vi "BallPositionTracking.vi"(8 "error in (no error)":errorcluster, 9 "Tracking treshold":i32=40, 10 "Circles Data":T2(array[cluster]), 11 "Screen Dimensions":cluster{"x":i32, "y":i32}) -> (0 "error out":errorcluster, 1 "maxDistance":i32, 2 "Ball Tracking Position Data":T1, 3 "Speed":i32, 5 "OOB":bool)   [LabVIEW 2015]
uses:
  <vilib>/vision/NI_Vision_Development_Module.lvlib
  <vilib>/Analysis/NI_AALPro.lvlib
panel:
  # "Input"
  # "Output"
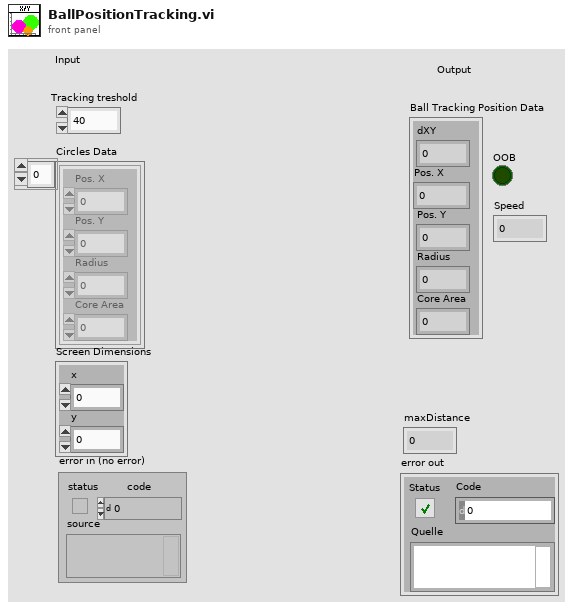
[diagram p1: front panel]
types:
  T1 = cluster{"dXY":i32, "Pos. X":i32, "Pos. Y":i32, "Radius":i32, "Core Area":i32}
  T2 = cluster{"Pos. X":i32, "Pos. Y":i32, "Radius":i32, "Core Area":i32}[]
  T3 = cluster{"dXY":i32, "Pos. X":i32, "Pos. Y":i32, "Radius":i32, "Core Area":i32}[]
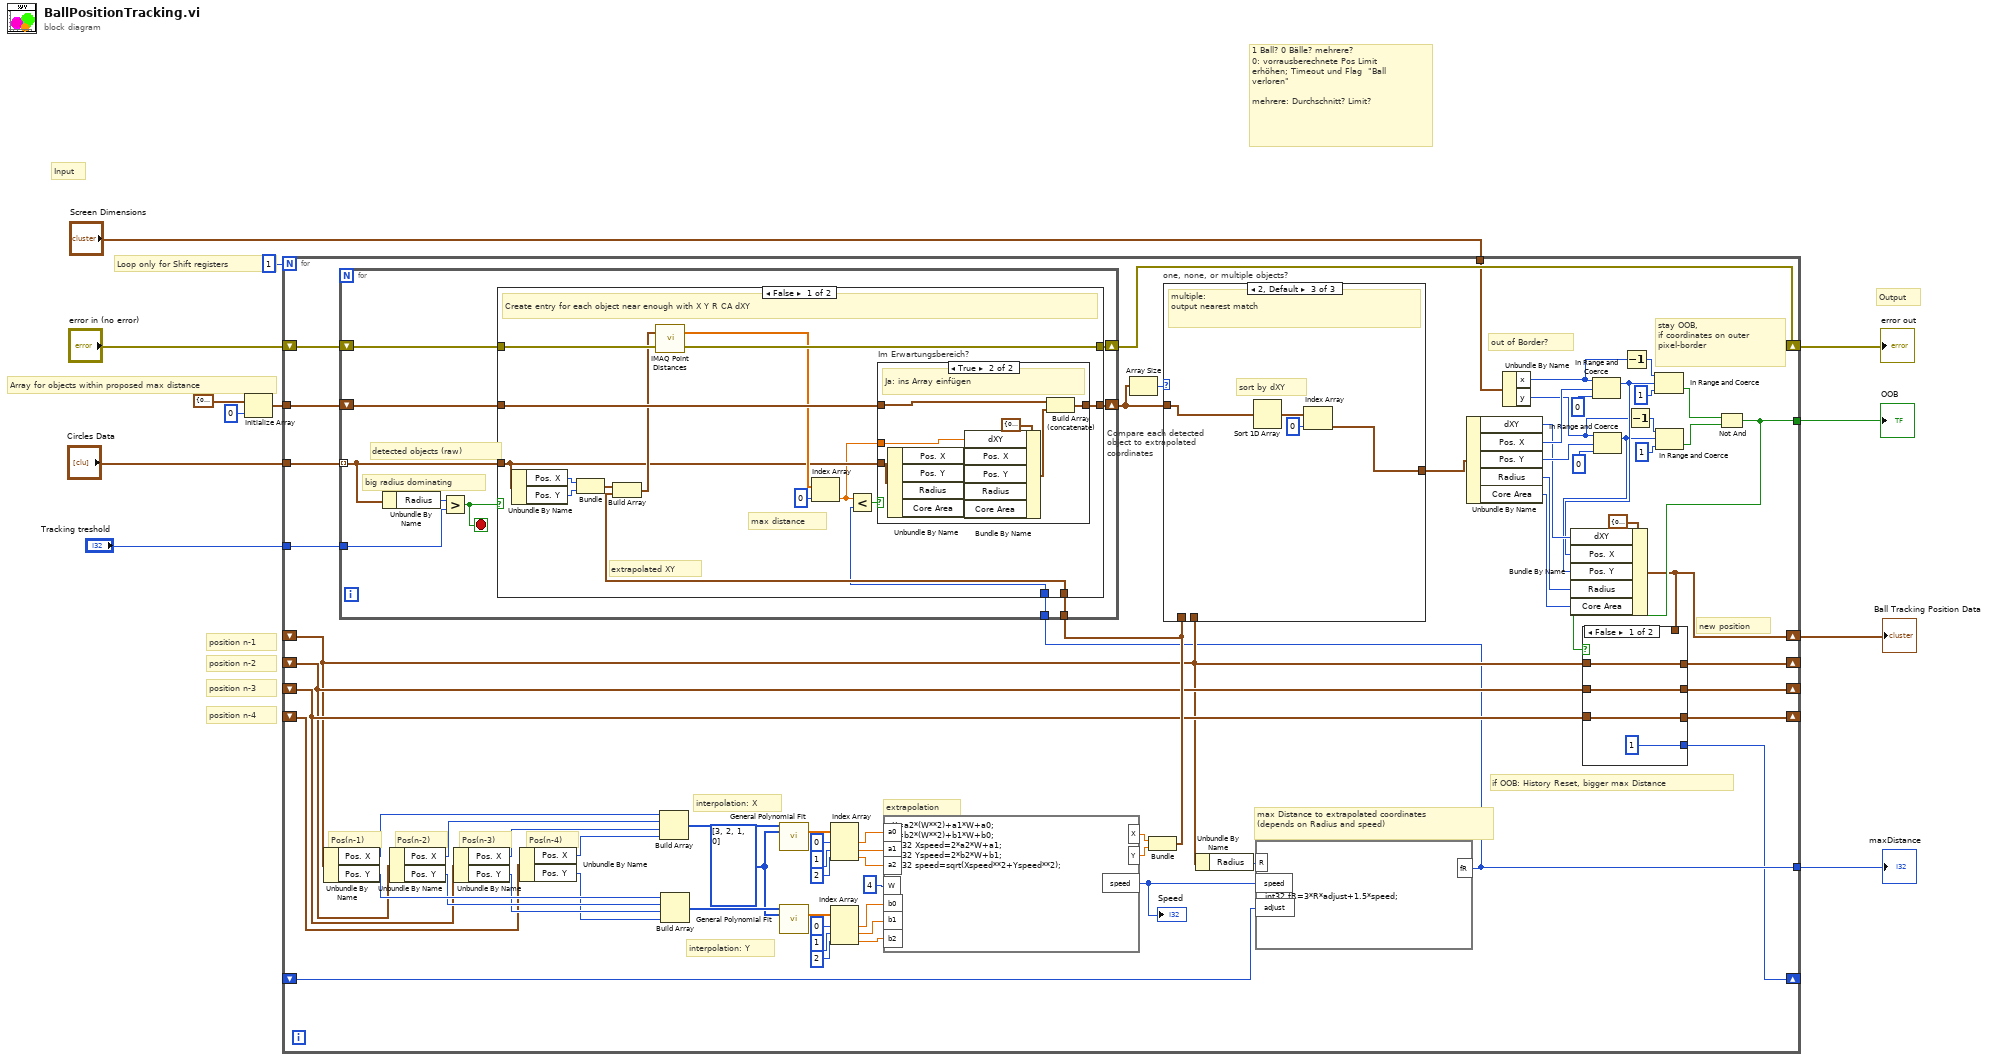
[diagram p0: block diagram]
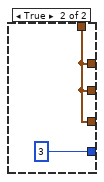
[diagram p2: hidden frame]
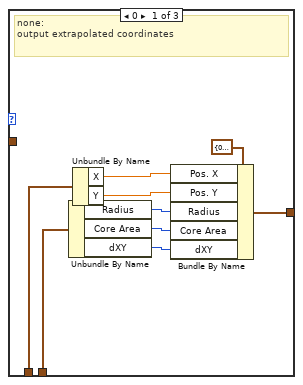
[diagram p3: hidden frame]
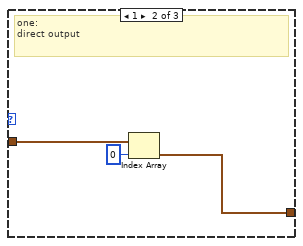
[diagram p4: hidden frame]
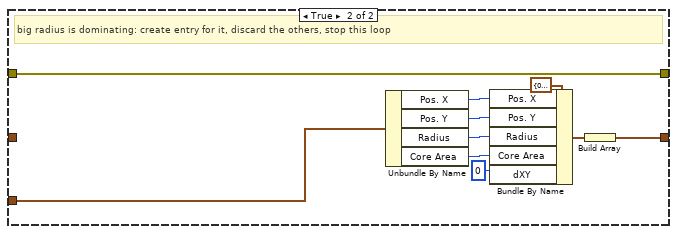
[diagram p6: hidden frame]
diagram:
  # "1 Ball? 0 Bälle? mehrere?\n0: vorrausberechnete Pos Limit erhöhen; Timeout und Flag  \"Ball verloren\"\n\nmehrere: Durchschnitt? Limit?"
  # "position n-4"
  # "Array for objects within proposed max distance"
  # "Loop only for Shift registers"
  # "position n-3"
  # "position n-2"
  # "position n-1"
  # "Output"
  # "Input"
  n1 = Initialize Array(T1 {"dXY"=0, "Pos. X"=0, "Pos. Y"=0, "Radius"=0, "Core Area"=0} ("Circles Data"), 0 ("Dimension")) -> (w8:T3)
  n2 = for {
    N: 1 -> [_]
    shift-right: [w30] -> w11
    shift-left: _ -> [w19]
    shift-right: [w80] -> w3
    shift-left: "error in (no error)" -> [w81]
    shift-right: [w34] -> _
    shift-left: _ -> [w35]
    shift-right: [w33] -> _
    shift-left: _ -> [w36]
    tunnel: w8 -> [w69]
    shift-right: [w32] -> _
    shift-left: _ -> [w49]
    tunnel: "Screen Dimensions" -> [w46]
    tunnel: [w31] -> w5
    tunnel: "Circles Data" -> [w82]
    tunnel: [w16] -> w4
    shift-right: [w14] -> _
    shift-left: _ -> [w15]
    tunnel: "Tracking treshold" -> [w13]
    w72 = i32[] [3, 2, 1, 0] ("X")
    # "new position"
    # "max Distance to extrapolated coordinates\n(depends on Radius and speed)"
    # "stay OOB,\nif coordinates on outer\npixel-border"
    # "if OOB: History Reset, bigger max Distance"
    # "out of Border?"
    # "Pos(n-4)"
    # "Pos(n-3)"
    # "Pos(n-2)"
    # "Pos(n-1)"
    # "extrapolation"
    # "interpolation: Y"
    # "interpolation: X"
    n3 = Unbundle By Name(w19) -> ("Pos. X"=w79:i32, "Pos. Y"=w76:i32)
    n4 = Unbundle By Name(w35) -> ("Pos. X"=w78:i32, "Pos. Y"=w75:i32)
    n5 = Unbundle By Name(w36) -> ("Pos. X"=w68:i32, "Pos. Y"=w74:i32)
    n6 = Unbundle By Name(w49) -> ("Pos. X"=w47:i32, "Pos. Y"=w48:i32)
    n7 = Build Array(w79, w78, w68, w47) -> (w77:i32[])
    n8 = Build Array(w76, w75, w74, w48) -> (w73:i32[])
    n9 = call <vilib>:"General Polynomial Fit.vi"("Y"=w77, "X"=w72) -> ("Polynomial Coefficients"=w54:dbl[])  [unwired: 10 in, 3 out]
    n10 = call <vilib>:"General Polynomial Fit.vi"("Y"=w73, "X"=w72) -> ("Polynomial Coefficients"=w64:dbl[])  [unwired: 10 in, 3 out]
    n11 = Index Array(array=w54, index #1=0 ("Index"), index #2=1 ("Index"), index #3=2 ("Index")) -> (element #1=w53:dbl, element #2=w52:dbl, element #3=w51:dbl)
    n12 = Index Array(array=w64, index #1=0 ("Index"), index #2=1 ("Index"), index #3=2 ("Index")) -> (element #1=w60:dbl, element #2=w59:dbl, element #3=w58:dbl)
    n13 = formula code="X=a2*(W**2)+a1*W+a0;\nY=b2*(W**2)+b1*W+b0;\nint32 Xspeed=2*a2*W+a1;\nint32 Yspeed=2*b2*W+b1;\nint32 speed=sqrt(Xspeed**2+Yspeed**2);"("a1"=w52, "b2"=w58, "a0"=w53, "b0"=w60, "b1"=w59, "a2"=w51, "W"=4 ("Eingangsvariable")) -> ("X"=w71:dbl, "Y"=w70:dbl, "speed"=w18:i32)
    "Speed" <- w18
    n14 = Bundle("X"=w71, "Y"=w70) -> (w65:cluster{"X":dbl, "Y":dbl})  [unwired: 1 in]
    n15 = Unbundle By Name(w19) -> ("Radius"=w17:i32)
    n16 = formula code="int32 fR=3*R*adjust+1.5*speed;"("R"=w17, "speed"=w18, "adjust"=w15) -> ("fR"=w16:i32)
    n17 = for {
      tunnel: w82 -> [w113] mode=indexing
      shift-right: [w109] -> w80
      shift-left: w81 -> [w110]
      tunnel: w65 -> [w111]
      shift-right: [w107] -> w66
      shift-left: w69 -> [w108]
      tunnel: w16 -> [w106]
      tunnel: w13 -> [w105]
      stop <- w112 stop-if-true
      # "detected objects (raw)"
      # "big radius dominating"
      n18 = Unbundle By Name(w113) -> ("Radius"=w114:i32)
      n19 = Greater?(x=w114, y=w105) -> (0:w112:bool)
      n20 = case "Compare each detected object to extrapolated coordinates" shown="False" w112 {
        tunnel: w113 -> [w118 w141]
        tunnel: w111 -> [w116 _]
        tunnel: w110 -> [w129 w150]
        tunnel: [w128 w150] -> w109
        tunnel: w108 -> [w124 _]
        tunnel: [w123 w142] -> w107
        tunnel: w106 -> [w115 _]
        frame False {
          # "max distance"
          # "extrapolated XY"
          # "Create entry for each object near enough with X Y R CA dXY"
          n21 = Unbundle By Name(w118) -> ("Pos. X"=w126:i32, "Pos. Y"=w125:i32)
          n22 = Bundle("Pos. X"=w126, "Pos. Y"=w125) -> (w127:cluster{"Pos. X":i32, "Pos. Y":i32})  [unwired: 1 in]
          n23 = Build Array(w127, w116) -> (w121:cluster{"X":dbl, "Y":dbl}[])
          n24 = call "IMAQ Point Distances"("Points"=w121, "error in (no error)"=w129) -> ("Distances"=w119:sgl[], "error out"=w128:errorcluster)  [unwired: 3 in]
          n25 = Index Array(array=w119, index=0 ("Index")) -> (element=w117:sgl)
          n26 = Less?(x=w117, y=w115) -> (x < y?=w122:bool)
          n27 = case "Im Erwartungsbereich?" shown="True" w122 {
            tunnel: w124 -> [w130 w140]
            tunnel: [w130 w137] -> w123
            tunnel: w118 -> [_ w139]
            tunnel: w117 -> [_ w131]
            frame False {
              # "Nein: nicht hinzufügen"
            }
            frame True {
              # "Ja: ins Array einfügen"
              n28 = Unbundle By Name(w139) -> ("Pos. X"=w135:i32, "Pos. Y"=w134:i32, "Radius"=w133:i32, "Core Area"=w132:i32)
              n29 = Bundle By Name(cluster=T1 {"dXY"=0, "Pos. X"=0, "Pos. Y"=0, "Radius"=0, "Core Area"=0} ("Circles Data"), "dXY"=w131, "Pos. X"=w135, "Pos. Y"=w134, "Radius"=w133, "Core Area"=w132) -> (w136:T1)
              n30 = Build Array (concatenate)(w140, w136) -> (w137:T3)
            }
          }
        }
        frame True {
          # "big radius is dominating: create entry for it, discard the others, stop this loop"
          n31 = Unbundle By Name(w141) -> ("Pos. X"=w148:i32, "Pos. Y"=w147:i32, "Radius"=w146:i32, "Core Area"=w145:i32)
          n32 = Bundle By Name(cluster=T1 {"dXY"=0, "Pos. X"=0, "Pos. Y"=0, "Radius"=0, "Core Area"=0} ("Circles Data"), "Pos. X"=w148, "Pos. Y"=w147, "Radius"=w146, "Core Area"=w145, "dXY"=0) -> (w143:T1)
          n33 = Build Array(w143) -> (w142:T3)
        }
      }
    }
    n34 = Array Size(array=w66) -> (size(s)=w67:i32)
    n35 = case "one, none, or multiple objects?" shown="2, Default" w67 {
      tunnel: w66 -> [_ w100 w104]
      tunnel: [w92 w98 w101] -> w41
      tunnel: w65 -> [w89 _ _]
      tunnel: w19 -> [w97 _ _]
      frame 0 {
        # "none:\noutput extrapolated coordinates"
        n36 = Unbundle By Name(w97) -> ("Radius"=w96:i32, "Core Area"=w95:i32, "dXY"=w90:i32)
        n37 = Unbundle By Name(w89) -> ("X"=w94:dbl, "Y"=w93:dbl)
        n38 = Bundle By Name(cluster=T1 {"dXY"=0, "Pos. X"=0, "Pos. Y"=0, "Radius"=0, "Core Area"=0} ("Circles Data"), "Pos. X"=w94, "Pos. Y"=w93, "Radius"=w96, "Core Area"=w95, "dXY"=w90) -> (w92:T1)
      }
      frame 1 {
        # "one:\ndirect output"
        n39 = Index Array(array=w100, index=0 ("Index")) -> (element=w98:T1)
      }
      frame 2, Default {
        # "sort by dXY"
        # "multiple:\noutput nearest match"
        n40 = Sort 1D Array(array=w104) -> (sorted array=w103:T3)
        n41 = Index Array(array=w103, index=0 ("Index")) -> (element=w101:T1)
      }
    }
    n42 = Unbundle By Name(w41) -> ("dXY"=w39:i32, "Pos. X"=w43:i32, "Pos. Y"=w42:i32, "Radius"=w38:i32, "Core Area"=w37:i32)
    n43 = Unbundle By Name(w46) -> ("x"=w27:i32, "y"=w23:i32)
    n44 = In Range and Coerce(upper limit=w27, x=w43, lower limit=0 ("Untergrenze")) -> (coerced(x)=w29:i32)  [unwired: 1 out]
    n45 = In Range and Coerce(upper limit=w23, x=w42, lower limit=0 ("Untergrenze")) -> (coerced(x)=w28:i32)  [unwired: 1 out]
    n46 = Bundle By Name(cluster=T1 {"dXY"=0, "Pos. X"=0, "Pos. Y"=0, "Radius"=0, "Core Area"=0} ("Circles Data"), "dXY"=w39, "Pos. X"=w29, "Pos. Y"=w28, "Radius"=w38, "Core Area"=w37) -> (w30:T1)
    n47 = Decrement(x=w27) -> (x-1=w26:i32)
    n48 = Decrement(x=w23) -> (x-1=w22:i32)
    n49 = In Range and Coerce(upper limit=w26, x=w29, lower limit=1 ("Untergrenze")) -> (In Range?=w25:bool)  [unwired: 1 out]
    n50 = In Range and Coerce(upper limit=w22, x=w28, lower limit=1 ("Untergrenze")) -> (In Range?=w24:bool)  [unwired: 1 out]
    n51 = Not And(1:w24, 2:w25) -> (0:w31:bool)
    n52 = case shown="False" w31 {
      tunnel: w19 -> [w86 _]
      tunnel: w36 -> [w84 _]
      tunnel: w35 -> [w85 _]
      tunnel: [w86 w88] -> w34
      tunnel: [w85 w88] -> w33
      tunnel: [w84 w88] -> w32
      tunnel: w30 -> [_ w88]
      tunnel: [1 3] -> w14
      frame False {
      }
      frame True {
      }
    }
  }
  "OOB" <- w5
  "Ball Tracking Position Data" <- w11
  "maxDistance" <- w4
  "error out" <- w3
